vi "剖面数据_bbe_NAQDO.vi"(0 "Tabe Name":string="剖面数据", 1 "data":T1={"时间"=timestamp(0 s since 1904-01-01), "测量模式"="水样测试", "数据类型"="N", "数据标识"="N", "湖面水深"=0.0, "缆绳下放长度"=0.0, "层数"=0, "row"=0, "水温"=0.0, "DO"=0.0, "饱和度"=0.0, "绿藻"=0.0, "蓝藻"=0.0, "硅甲藻"=0.0, "隐藻"=0.0, "黄色物质"=0.0, "总藻"=0.0, "透光率"=0.0, "水深"=0.0, "设置水深"=0.0}, 3 "错误输入（无错误）":errorcluster) -> (10 "错误输出":errorcluster)   [LabVIEW 2016]
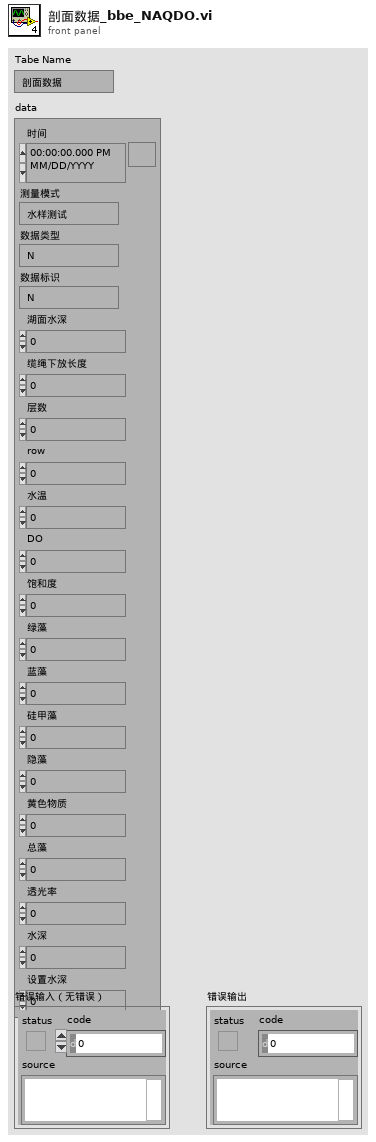
[diagram p1: front panel]
types:
  T1 = typedef "剖面数据_bbe_NAQDO.ctl" = cluster{"时间":timestamp, "测量模式":string, "数据类型":string, "数据标识":string, "湖面水深":sgl, "缆绳下放长度":sgl, "层数":u16, "row":u16, "水温":sgl, "DO":sgl, "饱和度":sgl, "绿藻":sgl, "蓝藻":sgl, "硅甲藻":sgl, "隐藻":sgl, "黄色物质":sgl, "总藻":sgl, "透光率":sgl, "水深":sgl, "设置水深":sgl}
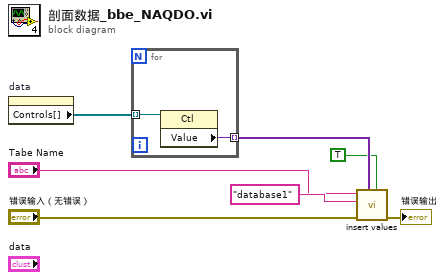
[diagram p0: block diagram]
diagram:
  n1 = property on="data" class="Clust (strict)"() -> ("Controls[]"=w7:refnum<vi>[])  [unwired: 2 in, 2 out]
  n2 = for {
    tunnel: w7 -> [w9] mode=indexing
    tunnel: [w8] -> w6 mode=indexing
    n3 = property class="Ctl"(reference=w9) -> ("Value"=w8:variant)  [unwired: 1 in, 2 out]
  }
  n4 = call "insert values.vi"("是否创建唯一键"=TRUE, "data"=w6, "错误输入（无错误）"="错误输入（无错误）", "database"="database1", "Tabe Name"="Tabe Name") -> ("错误输出"=→"错误输出":errorcluster)  [unwired: 6 in]
